vi "Element does not exist--error.vi"(4 "error in":errorcluster) -> (0 "error out":errorcluster)   [LabVIEW 2025]
doc: "Custom error -8001: This custom error signalizes that an element of a test project\ndoes not exist. This error is only relevant for testing, not for execution."
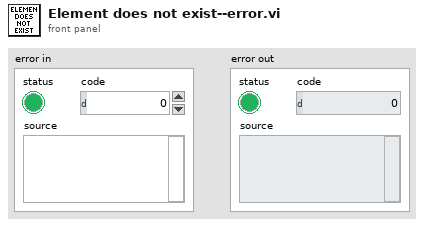
[diagram p1: front panel]
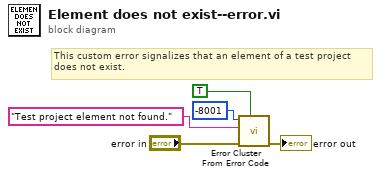
[diagram p0: block diagram]
diagram:
  # "This custom error signalizes that an element of a test project\ndoes not exist."
  n1 = call <vilib>:"Error Cluster From Error Code.vi"("show call chain? (False)"=TRUE, "error in (no error)"="error in", "error message (\"\")"="Test project element not found." ("format string"), "error code (0)"=-8001) -> ("error out"=→"error out":errorcluster)  [unwired: 5 in]
